vi "Configure Synthesizer Mode.vi"(8 "error in (no error)":errorcluster, 10 "Synthesizer Mode":enum16{"Normal", "Low Noise"}(ring), 11 "SigGen-8665B in":refnum<class "SigGen-8665B.lvclass">) -> (0 "error out":errorcluster, 3 "SigGen-8665B out":refnum<class "SigGen-8665B.lvclass">)   [LabVIEW 2020, in "SigGen-8665B.lvclass"]
uses:
  SigGen-8665B.lvclass
  C:/Sandbox/Git_Sandbox/WiSpry Test Framework source code (LV20)/WiSpry Test Framework/Instruments/Signal Generator/Signal Generator.lvclass
  C:/Sandbox/Git_Sandbox/WiSpry Test Framework source code (LV20)/WiSpry Test Framework/Instruments/Instrument.lvclass
  Signal Generator.lvclass/Signal Generator.ctl
  Instrument.lvclass/Instrument.ctl
  Signal Generator.lvclass
  Instrument.lvclass
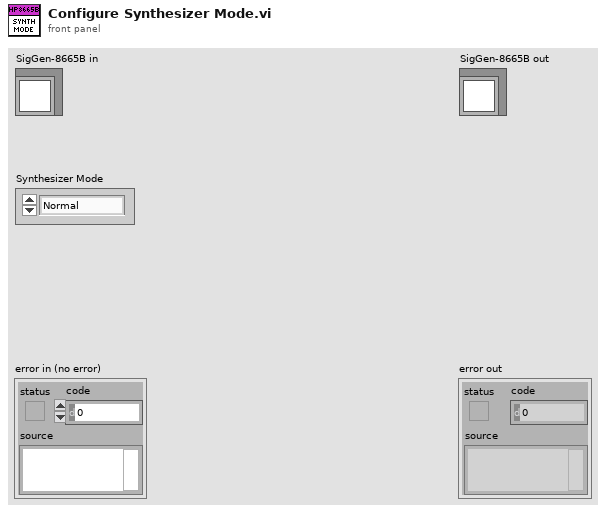
[diagram p1: front panel]
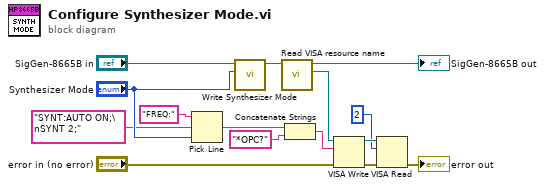
[diagram p0: block diagram]
diagram:
  n1 = Pick Line(string ("")="FREQ:", multi-line string="SYNT:AUTO ON;\nSYNT 2;", line index="Synthesizer Mode") -> (output string=w10:string)
  n2 = call "Write Synthesizer Mode.vi"("Synthesizer Mode"="Synthesizer Mode", "Signal Generator in"="SigGen-8665B in") -> ("Signal Generator out"=w14:refnum<class "SigGen-8665B.lvclass">)  [unwired: 9 in]
  n3 = call "Read VISA resource name.vi"("Instrument in"=w14) -> ("VISA resource name"=w8:refnum<visa-resource-name>, "Instrument out"=→"SigGen-8665B out":refnum<class "SigGen-8665B.lvclass">)  [unwired: 9 in]
  n4 = Concatenate Strings(w10, "*OPC?" ("string")) -> (w6:string)
  n5 = VISA Write(VISA resource name=w8, write buffer=w6, error in (no error)="error in (no error)") -> (VISA resource name out=w3:refnum<visa-resource-name>, error out=w4:errorcluster)  [unwired: 1 out]
  n6 = VISA Read(VISA resource name=w3, byte count=u32 2, error in (no error)=w4) -> (error out=→"error out":errorcluster)  [unwired: 3 out]
